vi "send.vi"(7 "condition":bool, 8 "error in (no error)":errorcluster, 10 "input":string, 11 "port":refnum<visa-resource-name>) -> (0 "error out":errorcluster, 2 "condition":bool, 3 "VISA resource name":refnum<visa-resource-name>)   [LabVIEW 2012]
uses:
  <vilib>/Instr/_visa.llb/VISA Configure Serial Port (Instr).vi
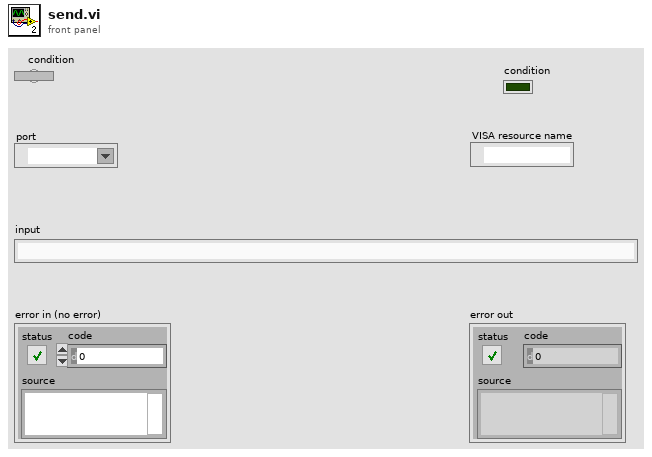
[diagram p1: front panel]
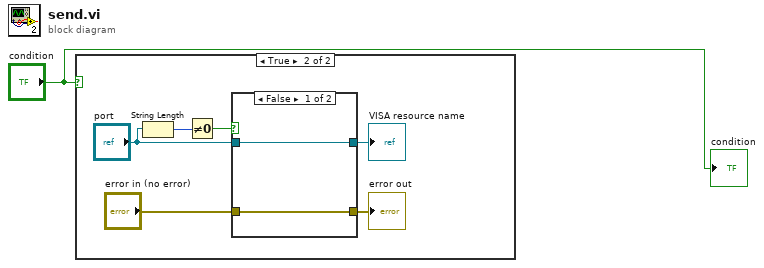
[diagram p0: block diagram]
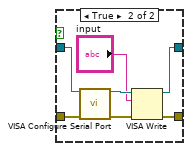
[diagram p3: hidden frame]
diagram:
  n1 = case shown="True" "condition" {
    frame False {
    }
    frame True {
      n2 = String Length(string="port") -> (length=w7:i32)
      n3 = Not Equal To 0?(x=w7) -> (x != 0?=w6:bool)
      n4 = case shown="False" w6 {
        tunnel: "port" -> [w9 w16]
        tunnel: [w9 w12] -> w4
        tunnel: "error in (no error)" -> [w8 w11]
        tunnel: [w8 w10] -> w2
        frame False {
        }
        frame True {
          n5 = call-poly "VISA Configure Serial Port"("VISA resource name"=w16, "error in (no error)"=w11) -> ("VISA resource name out"=w15:refnum<visa-resource-name>, "error out"=w14:errorcluster)  [unwired: 12 in]
          n6 = VISA Write(VISA resource name=w15, write buffer="input", error in (no error)=w14) -> (VISA resource name out=w12:refnum<visa-resource-name>, error out=w10:errorcluster)  [unwired: 1 out]
        }
      }
      "VISA resource name" <- w4
      "error out" <- w2
    }
  }
  "condition" <- "condition"
